vi "Save_Time_Traces_low.vi"(0 "Data Type":T1, 1 "Full Header Info?":bool, 2 "Put each block into separate file":bool, 3 "Precision":i16=2, 7 "Data to save":i32[](array[ring])=[1] items=["LDA (V)", "LDA (U)", "Save Nothing"], 9 "File Extension":string=".xls", 12 "Leave space between blocks?":bool, 13 "Time Series":enum16{"Milliseconds", "Seconds"}(ring), 14 "Separation Character":string="\t") -> ()   [LabVIEW 2010]
uses:
  Controls/Instrument_Array.ctl
  Globals/Meas_global.vi
  Acquisition/PWA/PWAtasksGLOBAL.vi
  Globals/Plug_in_data_global.vi
  Globals/LDA_meas_global_1.vi
panel:
  # "Run this VI to update the channel names"
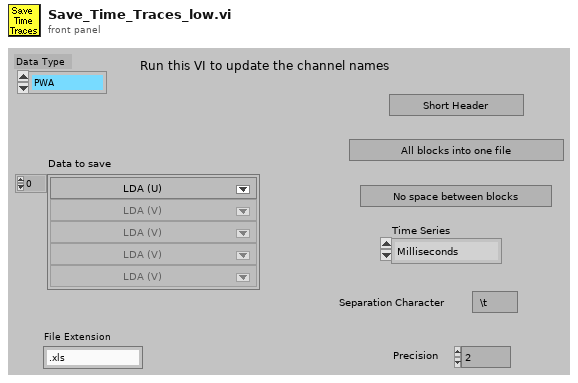
[diagram p1: front panel]
types:
  T1 = typedef "Instrument_Array.ctl" = enum16{"PWA", "LDA", "Analogue"}
  T2 = typedef "Analysis_info_cluster.ctl" = cluster{"Colour":u32, "Inst type":T3, "Inst name":string, "Symbol":string, "Code name":string, "Extra Info":string, "Inst Array":T1, "Index":i32, "Voltage Index":i32, "Extra Titles":string[], "Extra Values":string[]}
  T3 = typedef "Inst_type.ctl" = enum16{"Propeller anemometer", "Raw voltage", "Pressure Transducer", "Pitot-static tube", "Preston tube", "Hot wire", "Cross wire 1", "Cross wire 2", "Generic Linear", "Generic Polynomial", "Generic BackPoly", "Fast FID", "Thermocouple", "Cold wire", "Pulsed Wire", "LDA Vel", "LDA Tran time", "LDA Arr time"}
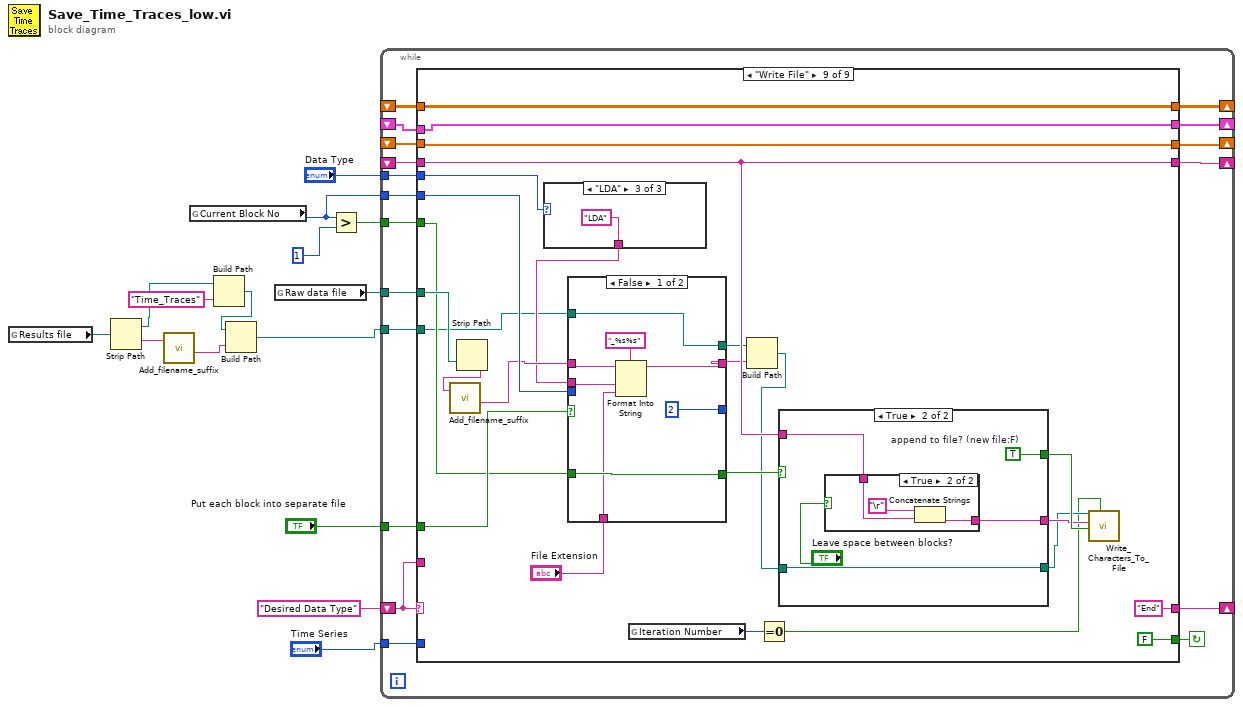
[diagram p0: block diagram]
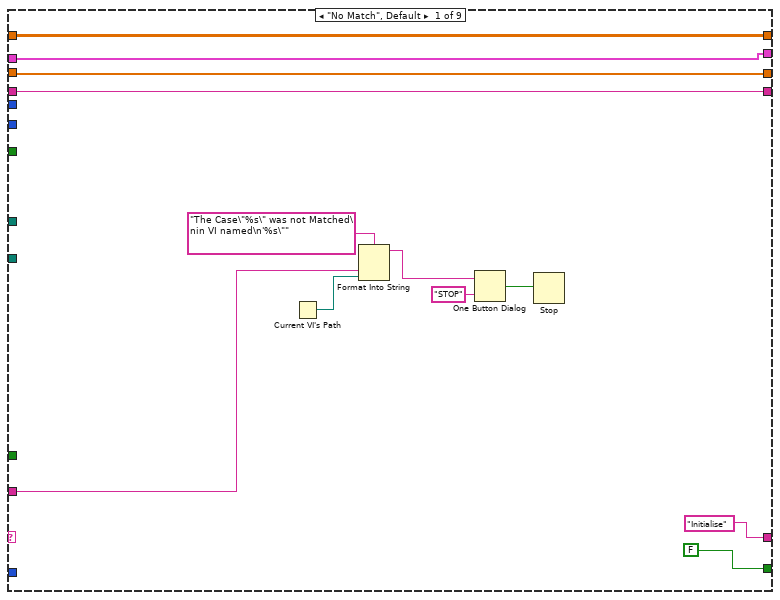
[diagram p2: hidden frame]
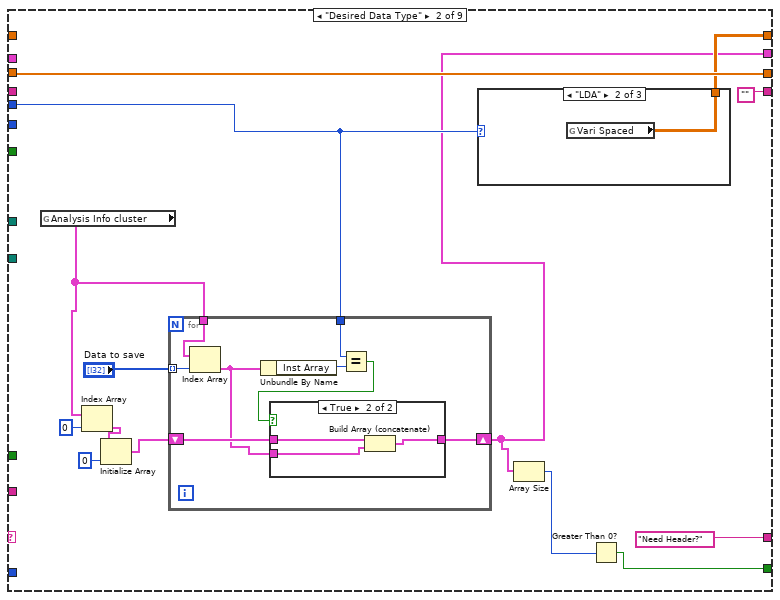
[diagram p3: hidden frame]
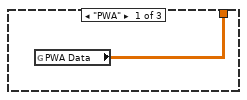
[diagram p5: hidden frame]
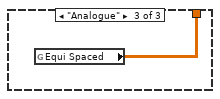
[diagram p6: hidden frame]
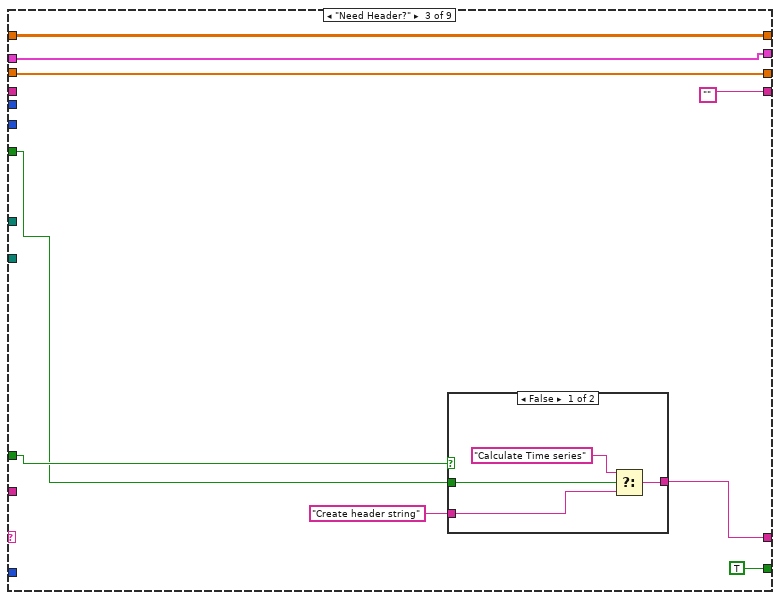
[diagram p7: hidden frame]
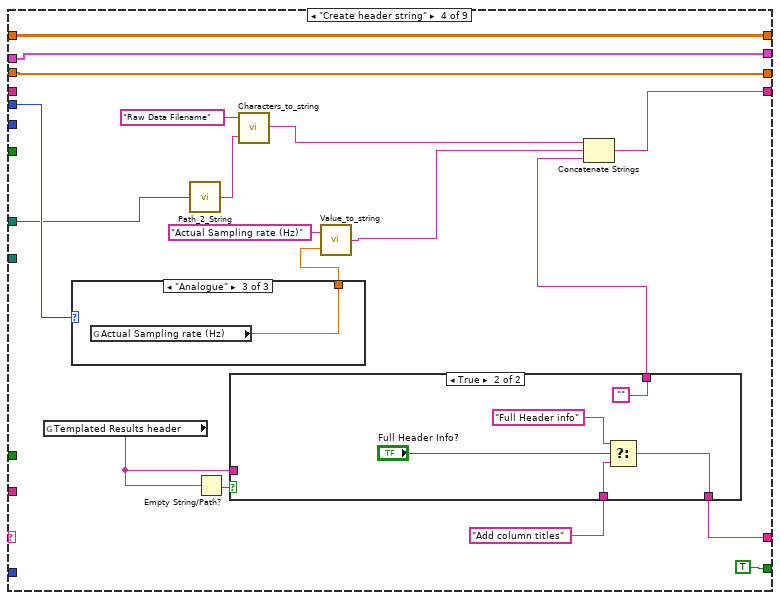
[diagram p9: hidden frame]
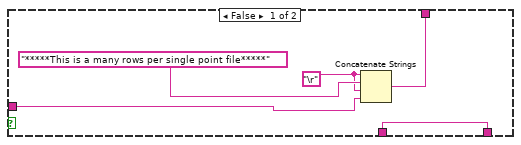
[diagram p10: hidden frame]
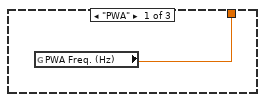
[diagram p11: hidden frame]
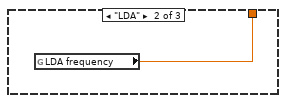
[diagram p12: hidden frame]
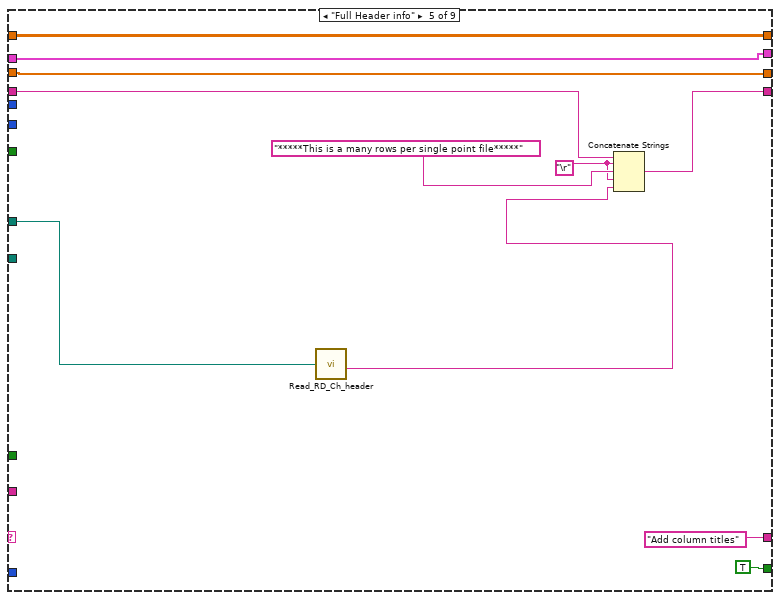
[diagram p13: hidden frame]
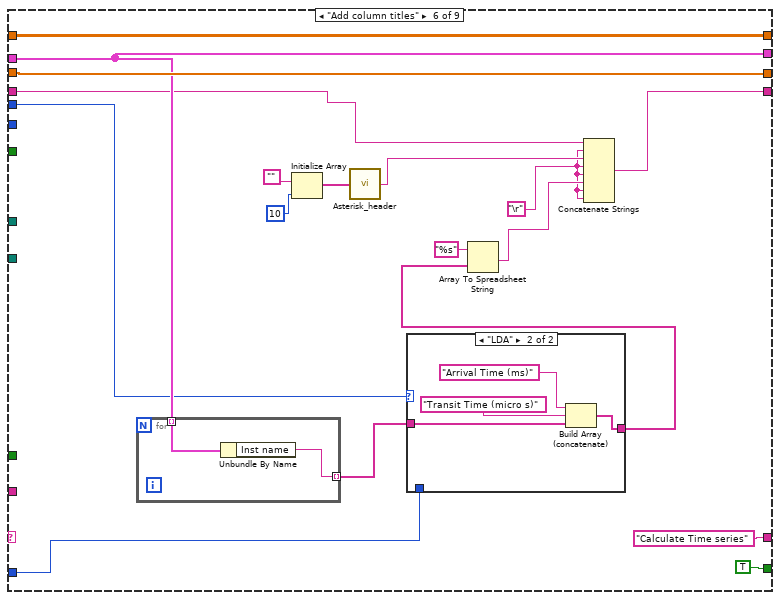
[diagram p14: hidden frame]
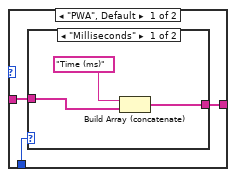
[diagram p15: hidden frame]
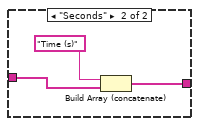
[diagram p16: hidden frame]
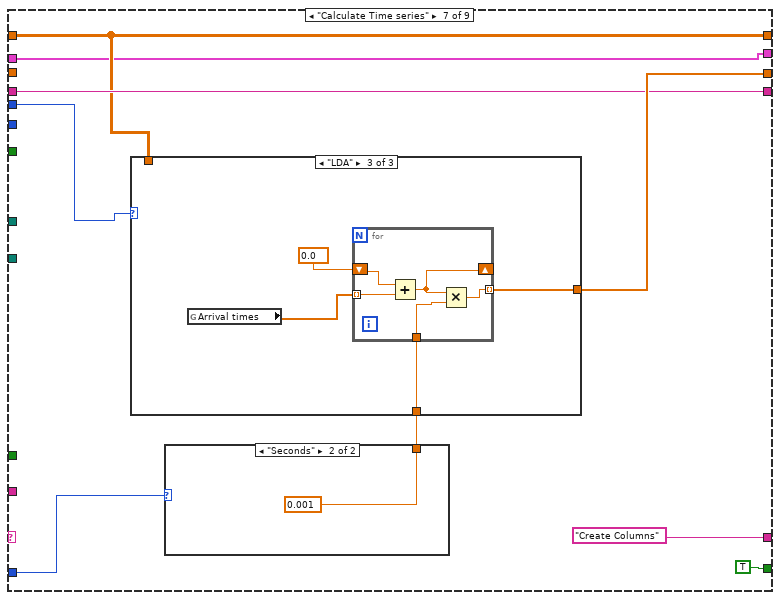
[diagram p17: hidden frame]
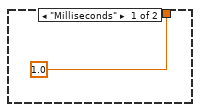
[diagram p18: hidden frame]
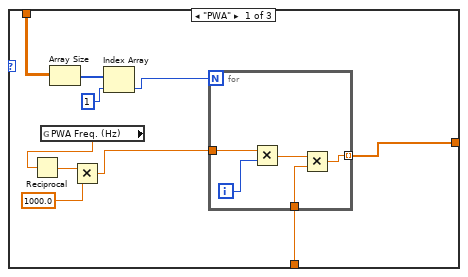
[diagram p19: hidden frame]
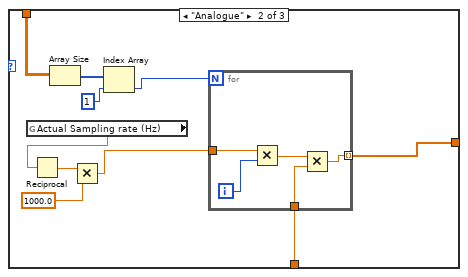
[diagram p20: hidden frame]
diagram:
  n1 = global read "Meas_global.vi" "Results file"() -> (w7:path)
  n2 = Strip Path(path=w7) -> (stripped path=w3:path, name=w6:string)
  n3 = call "Add_filename_suffix.vi"("Filename"=w6) -> ("Base name"=w5:string)  [unwired: 1 in, 3 out]
  n4 = global read "Meas_global.vi" "Current Block No"() -> (w11:i32)
  n5 = Build Path(base path=w3, name or relative path="Time_Traces") -> (appended path=w1:path)
  n6 = Build Path(base path=w1, name or relative path=w5) -> (appended path=w4:path)
  n7 = global read "Meas_global.vi" "Raw data file"() -> (w8:path)
  n8 = Greater?(x=w11, y=1) -> (0:w12:bool)
  n9 = while {
    shift-left: "Desired Data Type" -> [w31]
    shift-right: [w32] -> _
    shift-right: [w28] -> _
    shift-left: _ -> [w27]
    tunnel: "Put each block into separate file" -> [w30]
    tunnel: w8 -> [w29]
    tunnel: w12 -> [w26]
    shift-right: [w25] -> _
    shift-left: _ -> [w24]
    tunnel: w11 -> [w23]
    shift-right: [w22] -> _
    shift-left: _ -> [w21]
    tunnel: "Time Series" -> [w20]
    tunnel: "Data Type" -> [w19]
    shift-right: [w18] -> _
    shift-left: _ -> [w17]
    tunnel: w4 -> [w16]
    stop <- w33 continue-if-true
    n10 = case shown="\"Write File\"" w31 {
      tunnel: [FALSE w47 TRUE TRUE TRUE TRUE TRUE TRUE FALSE] -> w33
      tunnel: ["Initialise" "Need Header?" w80 w90 "Add column titles" ("t") "Calculate Time series" ("t") "Create Columns" ("t") "Write File" "End" ("t")] -> w32
      tunnel: w31 -> [w40 _ _ _ _ _ _ _ _]
      tunnel: w30 -> [_ _ w79 _ _ _ _ _ w295]
      tunnel: w29 -> [_ _ _ w95 w121 _ _ _ w305]
      tunnel: [w37 "" "" w103 w122 w146 w169 w222 w301] -> w28
      tunnel: w27 -> [w37 _ _ _ w123 w137 w169 w224 w301]
      tunnel: w26 -> [_ _ w78 _ _ _ _ _ w291]
      tunnel: [w36 w58 w82 w102 w129 w144 w171 w216 w298] -> w25
      tunnel: w24 -> [w36 w58 w82 w102 w129 w144 _ w216 w298]
      tunnel: w23 -> [_ _ _ _ _ _ _ _ w297]
      tunnel: [w35 w57 w77 w99 w128 w142 w168 w220 w292] -> w22
      tunnel: w21 -> [w35 _ w77 w99 w128 w142 w168 w220 w292]
      tunnel: w20 -> [_ _ _ _ _ w131 w167 w219 _]
      tunnel: w19 -> [_ w54 _ w97 _ w134 w165 w215 w287]
      tunnel: [w34 w46 w75 w96 w126 w141 w164 w217 w288] -> w18
      tunnel: w17 -> [w34 _ w75 w96 w126 w141 w164 w217 w288]
      tunnel: w16 -> [_ _ _ _ _ _ _ _ w284]
      frame "No Match", Default {
        n11 = Current VI's Path() -> (path=w39:path)
        n12 = Format Into String(format string="The Case\"%s\" was not Matched\nin VI named\n'%s\"" ("Format String"), w40, w39) -> (resulting string=w43:string)  [unwired: 2 in, 1 out]
        n13 = One Button Dialog(message=w43, button name ("OK")="STOP") -> (true=w41:bool)
        n14 = Stop(stop? (T)=w41) -> ()
      }
      frame "Desired Data Type" {
        n15 = global read "Meas_global.vi" "Analysis Info cluster"() -> (w50:T2[])
        n16 = Index Array(array=w50, index=0) -> (element=w51:T2)
        n17 = Initialize Array(w51, 0 ("dimension size")) -> (w53:T2[])
        n18 = for {
          tunnel: w50 -> [w67]
          tunnel: "Data to save" -> [w66] mode=indexing
          tunnel: w54 -> [w64]
          shift-right: [w60] -> w46
          shift-left: w53 -> [w62]
          n19 = Index Array(array=w67, index=w66) -> (element=w61:T2)
          n20 = Unbundle By Name(w61) -> ("Inst Array"=w65:T1)
          n21 = Equal?(x=w64, y=w65) -> (x = y?=w63:bool)
          n22 = case shown="True" w63 {
            tunnel: w62 -> [w68 w71]
            tunnel: w61 -> [_ w70]
            tunnel: [w68 w69] -> w60
            frame False {
            }
            frame True {
              n23 = Build Array (concatenate)(w71, w70) -> (w69:T2[])
            }
          }
        }
        n24 = case shown="\"LDA\"" w54 {
          tunnel: [w72 w73 w74] -> w57
          frame "PWA" {
            n25 = global read "PWAtasksGLOBAL.vi" "PWA Data"() -> (w72:dbl[][])
          }
          frame "LDA" {
            n26 = global read "Plug_in_data_global.vi" "Vari Spaced"() -> (w73:dbl[][])
          }
          frame "Analogue" {
            n27 = global read "Plug_in_data_global.vi" "Equi Spaced"() -> (w74:dbl[][])
          }
        }
        n28 = Array Size(array=w46) -> (size(s)=w48:i32)
        n29 = Greater Than 0?(x=w48) -> (x > 0?=w47:bool)
      }
      frame "Need Header?" {
        n30 = case shown="False" w79 {
          tunnel: [w87 w88] -> w80
          tunnel: w78 -> [w86 _]
          tunnel: "Create header string" -> [w84 w88]
          frame False {
            n31 = Select(t="Calculate Time series", s=w86, f=w84) -> (s? t:f=w87:string)
          }
          frame True {
          }
        }
      }
      frame "Create header string" {
        n32 = global read "Plug_in_data_global.vi" "Templated Results header"() -> (w92:string)
        n33 = case shown="\"Analogue\"" w97 {
          tunnel: [w117 w118 w119] -> w98
          frame "PWA" {
            n34 = global read "PWAtasksGLOBAL.vi" "PWA Freq. (Hz)"() -> (w117:dbl)
          }
          frame "LDA" {
            n35 = global read "Meas_global.vi" "LDA frequency"() -> (w118:dbl)
          }
          frame "Analogue" {
            n36 = global read "Meas_global.vi" "Actual Sampling rate (Hz)"() -> (w119:dbl)
          }
        }
        n37 = call "Path_2_String.vi"("Real Path"=w95) -> ("Path String"=w94:string)
        n38 = Empty String/Path?(string/path=w92) -> (empty?=w93:bool)
        n39 = case shown="True" w93 {
          tunnel: w92 -> [w109 _]
          tunnel: "Add column titles" ("t") -> [w108 w114]
          tunnel: [w108 w113] -> w90
          tunnel: [w107 ""] -> w89
          frame False {
            w110 = "\r"
            n40 = Concatenate Strings(w110, "*****This is a many rows per single point file*****", w110, w109) -> (w107:string)
          }
          frame True {
            n41 = Select(t="Full Header info", s="Full Header Info?", f=w114) -> (s? t:f=w113:string)
          }
        }
        n42 = call "Characters_to_string.vi"("Characters to write"=w94, "Label for characters"="Raw Data Filename") -> ("Output string"=w105:string)
        n43 = call "Value_to_string.vi"("Value"=w98, "Label for value"="Actual Sampling rate (Hz)") -> ("Output string"=w100:string)  [unwired: 1 in]
        n44 = Concatenate Strings(w105, w100, w89) -> (w103:string)
      }
      frame "Full Header info" {
        w124 = "\r"
        n45 = call "Read_RD_Ch_header.vi"("Raw data file"=w121) -> ("Ch string"=w120:string)  [unwired: 3 out]
        n46 = Concatenate Strings(w123, w124, "*****This is a many rows per single point file*****", w124, w120) -> (w122:string)
      }
      frame "Add column titles" {
        w135 = "\r"
        n47 = for {
          tunnel: [w162] -> w133 mode=indexing
          tunnel: w141 -> [w163] mode=indexing
          n48 = Unbundle By Name(w163) -> ("Inst name"=w162:string)
        }
        n49 = Initialize Array("", 10) -> (w138:string[])
        n50 = call "Asterisk_header.vi"("Channel names"=w138) -> ("Header string"=w136:string)
        n51 = case shown="\"LDA\"" w134 {
          tunnel: w133 -> [w151 w159]
          tunnel: [w150 w158] -> w132
          tunnel: w131 -> [w149 _]
          frame "PWA", Default {
            n52 = case shown="\"Milliseconds\"" w149 {
              tunnel: w151 -> [w154 w157]
              tunnel: [w153 w156] -> w150
              frame "Milliseconds" {
                n53 = Build Array (concatenate)("Time (ms)", w154) -> (w153:string[])
              }
              frame "Seconds" {
                n54 = Build Array (concatenate)("Time (s)", w157) -> (w156:string[])
              }
            }
          }
          frame "LDA" {
            n55 = Build Array (concatenate)("Arrival Time (ms)", "Transit Time (micro s)", w159) -> (w158:string[])
          }
        }
        n56 = Array To Spreadsheet String(array=w132, 3:"%s" ("format string")) -> (spreadsheet string=w143:string)  [unwired: 1 out]
        n57 = Concatenate Strings(w137, w135, w136, w135, w135, w143, w135, w135) -> (w146:string)
      }
      frame "Calculate Time series" {
        n58 = case shown="\"Seconds\"" w167 {
          tunnel: [1.0 0.001] -> w166
          frame "Milliseconds" {
          }
          frame "Seconds" {
          }
        }
        n59 = case shown="\"LDA\"" w165 {
          tunnel: [w175 w190 w205] -> w171
          tunnel: w168 -> [w180 w195 _]
          tunnel: w166 -> [w177 w191 w206]
          frame "PWA" {
            n60 = global read "PWAtasksGLOBAL.vi" "PWA Freq. (Hz)"() -> (w176:dbl)
            n61 = Reciprocal(x=w176) -> (1/x=w184:dbl)
            n62 = Array Size(array=w180) -> (size(s)=w181:i32[])
            n63 = Multiply(x=w184, y=1000.0) -> (x*y=w182:dbl)
            n64 = Index Array(array=w181, index=1) -> (element=w178:i32)
            n65 = for {
              N: w178 -> [_]
              tunnel: w182 -> [w188]
              tunnel: [w186] -> w175 mode=indexing
              tunnel: w177 -> [w185]
              i -> [w189]
              n66 = Multiply(x=w188, y=w189) -> (x*y=w187:dbl)
              n67 = Multiply(x=w187, y=w185) -> (x*y=w186:dbl)
            }
          }
          frame "Analogue" {
            n68 = global read "Meas_global.vi" "Actual Sampling rate (Hz)"() -> (w192:dbl)
            n69 = Reciprocal(x=w192) -> (1/x=w199:dbl)
            n70 = Array Size(array=w195) -> (size(s)=w196:i32[])
            n71 = Multiply(x=w199, y=1000.0) -> (x*y=w197:dbl)
            n72 = Index Array(array=w196, index=1) -> (element=w193:i32)
            n73 = for {
              N: w193 -> [_]
              tunnel: w197 -> [w203]
              tunnel: [w201] -> w190 mode=indexing
              tunnel: w191 -> [w200]
              i -> [w204]
              n74 = Multiply(x=w203, y=w204) -> (x*y=w202:dbl)
              n75 = Multiply(x=w202, y=w200) -> (x*y=w201:dbl)
            }
          }
          frame "LDA" {
            n76 = global read "LDA_meas_global_1.vi" "Arrival times"() -> (w208:dbl[])
            n77 = for {
              shift-right: [w211] -> _
              shift-left: 0.0 -> [w213]
              tunnel: w208 -> [w212] mode=indexing
              tunnel: [w210] -> w205 mode=indexing
              tunnel: w206 -> [w209]
              n78 = Add(x=w213, y=w212) -> (x+y=w211:dbl)
              n79 = Multiply(x=w211, y=w209) -> (x*y=w210:dbl)
            }
          }
        }
      }
      frame "Create Columns" {
        n80 = Array Size(array=w217) -> (size(s)=w227:i32)
        n81 = Decrement(x=w227) -> (x-1=w228:i32)
        n82 = global read "LDA_meas_global_1.vi" "Transit times"() -> (w214:dbl[])
        n83 = for {
          shift-right: [w245] -> w223
          shift-left: "" -> [w240]
          tunnel: "Separation Character" -> [w231]
          tunnel: w217 -> [w235]
          tunnel: w220 -> [w243]
          tunnel: w228 -> [w239]
          tunnel: w216 -> [w237] mode=indexing
          tunnel: w219 -> [w236]
          tunnel: w215 -> [w234]
          tunnel: w214 -> [w233]
          i -> [w232]
          n84 = case shown="\"Milliseconds\"" w236 {
            tunnel: [w257 w261] -> w230
            tunnel: w231 -> [w256 w260]
            tunnel: w237 -> [w255 w259]
            frame "Seconds" {
              n85 = Format Into String(format string="%.4f%s", w255, w256) -> (resulting string=w257:string)  [unwired: 2 in, 1 out]
            }
            frame "Milliseconds" {
              n86 = Format Into String(format string="%.2f%s", w259, w260) -> (resulting string=w261:string)  [unwired: 2 in, 1 out]
            }
          }
          n87 = Index Array(array=w243, index (col)=w232) -> (element=w242:dbl[])  [unwired: 1 in]
          n88 = case shown="\"LDA\"" w234 {
            tunnel: w233 -> [_ w253]
            tunnel: w232 -> [_ w252]
            tunnel: w231 -> [_ w249]
            tunnel: [w246 w248] -> w229
            tunnel: w230 -> [w246 w247]
            frame "PWA", Default {
            }
            frame "LDA" {
              n89 = Index Array(array=w253, index=w252) -> (element=w250:dbl)
              n90 = Format Into String(format string="%.2f%s", initial string=w247, w250, w249) -> (resulting string=w248:string)  [unwired: 1 in, 1 out]
            }
          }
          n91 = for {
            shift-right: [w271] -> w241
            shift-left: w229 -> [w273]
            tunnel: w231 -> [w270]
            tunnel: w242 -> [w269]
            tunnel: w239 -> [w266]
            tunnel: "Precision" -> [w264]
            tunnel: w235 -> [w263] mode=indexing
            i -> [w267]
            n92 = Unbundle By Name(w263) -> ("Index"=w262:i32)
            n93 = Index Array(array=w269, index=w262) -> (element=w268:dbl)
            n94 = Equal?(x=w267, y=w266) -> (x = y?=w265:bool)
            n95 = Number To Fractional String(number=w268, precision (6)=w264) -> (F-format string=w272:string)  [unwired: 2 out]
            n96 = case shown="True" w265 {
              tunnel: w273 -> [w277 w280]
              tunnel: w272 -> [w276 w279]
              tunnel: [w275 w278] -> w271
              tunnel: w270 -> [w274 _]
              frame False {
                n97 = Concatenate Strings(w277, w276, w274) -> (w275:string)
              }
              frame True {
                n98 = Concatenate Strings(w280, w279) -> (w278:string)
              }
            }
          }
          n99 = Concatenate Strings(w240, w241, "\r") -> (w245:string)
        }
        n100 = Concatenate Strings(w224, w223) -> (w222:string)
      }
      frame "Write File" {
        n101 = Strip Path(path=w305) -> (name=w289:string)  [unwired: 1 out]
        n102 = call "Add_filename_suffix.vi"("Filename"=w289) -> ("Base name"=w290:string)  [unwired: 1 in, 3 out]
        n103 = case shown="\"LDA\"" w287 {
          tunnel: ["PWA" "AN" "LDA"] -> w286
          frame "PWA" {
          }
          frame "Analogue" {
          }
          frame "LDA" {
          }
        }
        n104 = case shown="False" w295 {
          tunnel: w290 -> [w311 w322]
          tunnel: w297 -> [_ w319]
          tunnel: [w310 w325] -> w296
          tunnel: w291 -> [w316 _]
          tunnel: [w316 FALSE] -> w294
          tunnel: [w315 w321] -> w293
          tunnel: w284 -> [w315 w323]
          tunnel: [2 ("y") 3 ("y")] -> _
          tunnel: w286 -> [w312 w318]
          tunnel: "File Extension" -> [w309 w317]
          frame False {
            n105 = Format Into String(format string="_%s%s", initial string=w311, w312, w309) -> (resulting string=w310:string)  [unwired: 1 in, 1 out]
          }
          frame True {
            n106 = Format Into String(format string="_%s_%d%s", initial string=w322, w318, w319, w317) -> (resulting string=w325:string)  [unwired: 1 in, 1 out]
            n107 = Build Path(base path=w323, name or relative path=w322) -> (appended path=w321:path)
          }
        }
        n108 = global read "Meas_global.vi" "Iteration Number"() -> (w282:i32)
        n109 = Build Path(base path=w293, name or relative path=w296) -> (appended path=w283:path)
        n110 = Equal To 0?(x=w282) -> (x = 0?=w281:bool)
        n111 = case shown="True" w294 {
          tunnel: [w327 w335] -> w303
          tunnel: w301 -> [w327 w334]
          tunnel: [w330 w333] -> w304
          tunnel: w283 -> [w329 w331]
          tunnel: [w328 w331] -> w302
          frame False {
            w330 = FALSE  # append to file? (new file:F)
            n112 = call "Create_directory_path.vi"("Path name"=w329) -> ("Path name Out"=w328:path)
          }
          frame True {
            w333 = TRUE  # append to file? (new file:F)
            n113 = case shown="True" "Leave space between blocks?" {
              tunnel: [w336 w339] -> w335
              tunnel: w334 -> [w336 w338]
              frame False {
              }
              frame True {
                n114 = Concatenate Strings("\r", w338) -> (w339:string)
              }
            }
          }
        }
        n115 = call "Write_Characters_To_File.vi"("file path (dialog if empty)"=w302, "advisory dialog? (display:T)"=w281, "character string"=w303, "append to file? (new file:F)"=w304) -> ()  [unwired: 1 in, 4 out]
      }
    }
  }
